vi "Clousure.vi"(8 "error in (no error)":errorcluster, 11 "ConcreteCreatorB in":refnum<class "ConcreteCreatorB.lvclass">) -> (0 "error out":errorcluster, 3 "ConcreteCreatorB out":refnum<class "ConcreteCreatorB.lvclass">)   [LabVIEW 2020, in "FactoryMethod.lvlib" / "ConcreteCreatorB.lvclass"]
uses:
  ConcreteCreatorB.lvclass
  Creator/Creator.lvclass
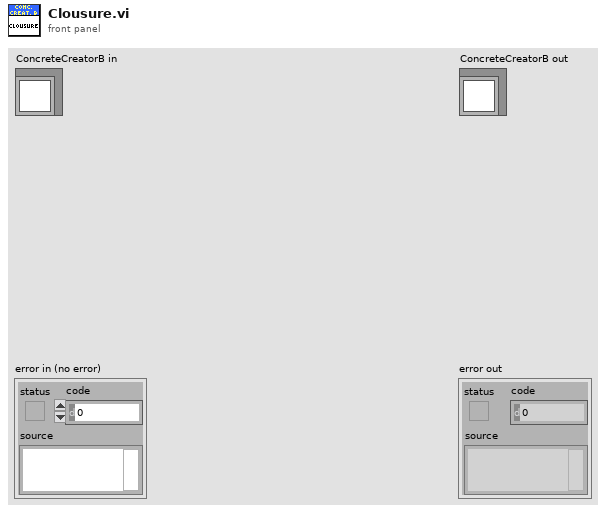
[diagram p1: front panel]
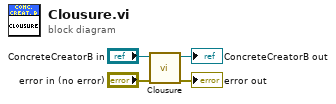
[diagram p0: block diagram]
diagram:
  n1 = call-parent "Clousure.vi"("error in (no error)"="error in (no error)", "Creator in"="ConcreteCreatorB in") -> ("error out"=→"error out":errorcluster, "Creator out"=→"ConcreteCreatorB out":refnum<class "ConcreteCreatorB.lvclass">)  [unwired: 8 in]
